vi "All_stats_labels.vi"() -> (0 "No of stats columns":i32[](array[numeric]), 3 "Stats labels":string[](array[string]))   [LabVIEW 2011]
uses:
  Controls/Inst_type.ctl
  Globals/Meas_global.vi
  Globals/Trav_pos_global.vi
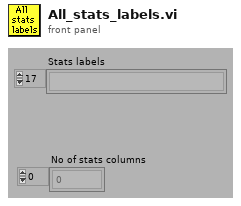
[diagram p1: front panel]
types:
  T1 = typedef "Tunnel_Coordinates.ctl" = enum16{"Work in Tunnel Coordinates", "Work in Model Coordinates"}
  T2 = typedef "Analysis_info_cluster.ctl" = cluster{"Colour":u32, "Inst type":T3, "Inst name":string, "Symbol":string, "Code name":string, "Extra Info":string, "Inst Array":T4, "Index":i32, "Voltage Index":i32, "Extra Titles":string[], "Extra Values":string[], "Eng Values":dbl[], "Time (ms)":dbl[], "TT / Voltage":dbl[], "U":dbl, "u^2":dbl, "u^3":dbl, "u^4":dbl, "Skew_u":dbl, "Kurt_u":dbl, "Sd Error in Mean":dbl, "% u'/U":dbl, "X":dbl, "Y":dbl, "Z":dbl, "Spectra":T5, "Autocorrelation":T5, "Timescale integral to 25%":dbl, "Sd Error in Variance":dbl, "Calib File":path, "Calib Constants":dbl[]}
  T3 = typedef "Inst_type.ctl" = enum16{"Propeller anemometer", "Raw voltage", "Pressure Transducer", "Pitot-static tube", "Preston tube", "Hot wire", "Cross wire 1", "Cross wire 2", "Generic Linear", "Generic Polynomial", "Generic BackPoly", "Fast FID", "Thermocouple", "Cold wire", "Pulsed Wire", "LDA Vel", "LDA Tran time", "LDA Arr time"}
  T4 = typedef "Instrument_Array.ctl" = enum16{"PWA", "LDA", "Analogue"}
  T5 = typedef "XY_Plot_Cluster.ctl" = cluster{"First Name":string, "Second Name":string, "X axis name":string, "Y axis name":string, "X array":dbl[], "Y array":dbl[]}
  T6 = typedef "Analysis_type_cluster.ctl" = cluster{"Analysis type":T7, "Indicies":i32[], "Name":string, "Inst Array":T4, "Info index":i32}
  T7 = typedef "Analysis_type_Enum.ctl" = enum16{"Slow Response", "Fast Response", "Weighted Fast Response", "Fast FID", "Weighted Fast FID", "Cross Wire", "Weighted Cross Wire", "Weighted LDA"}
  T8 = enum16{"Mean only", "2nd Order Stats", "4th Order Stats"}
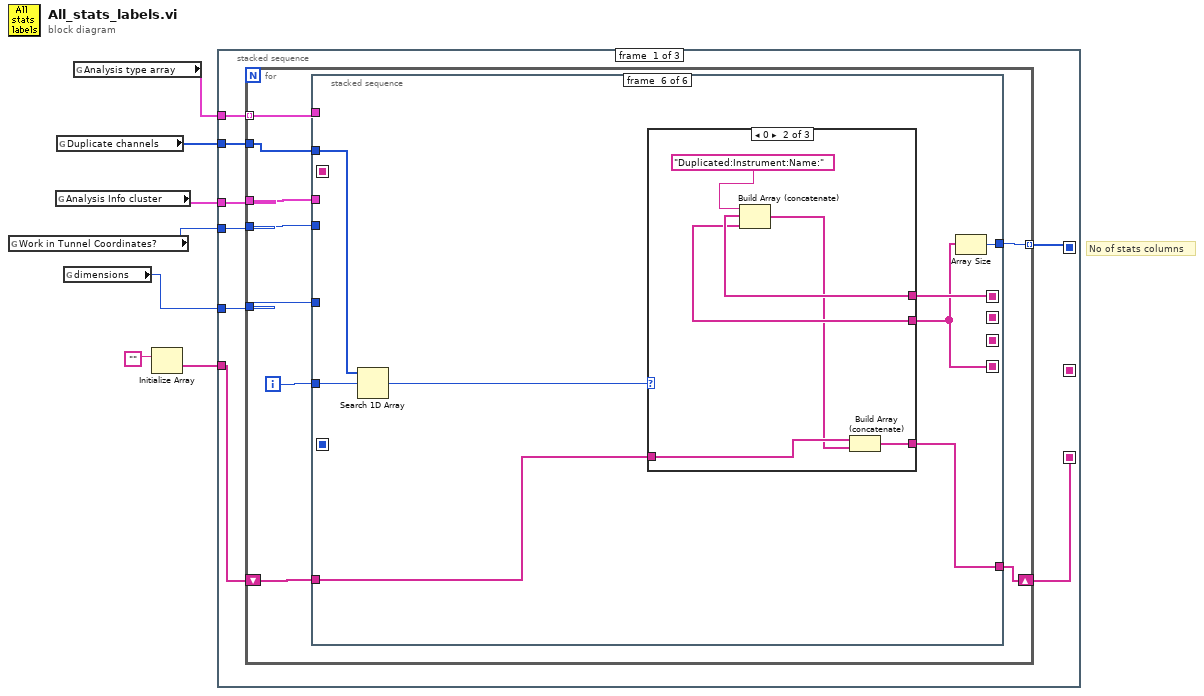
[diagram p0: block diagram]
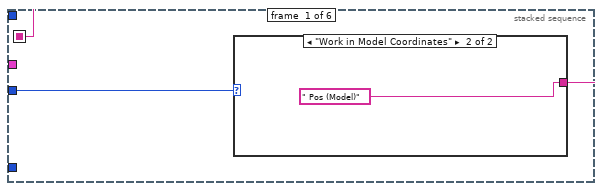
[diagram p2: hidden frame]
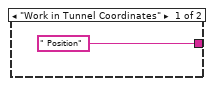
[diagram p3: hidden frame]
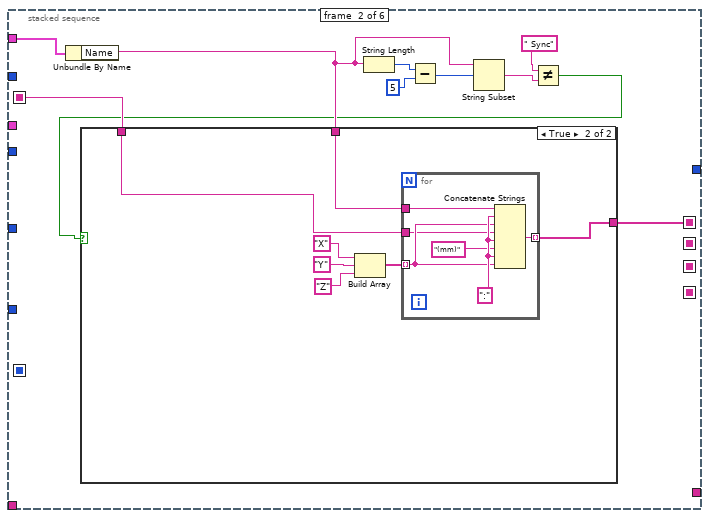
[diagram p4: hidden frame]
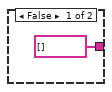
[diagram p5: hidden frame]
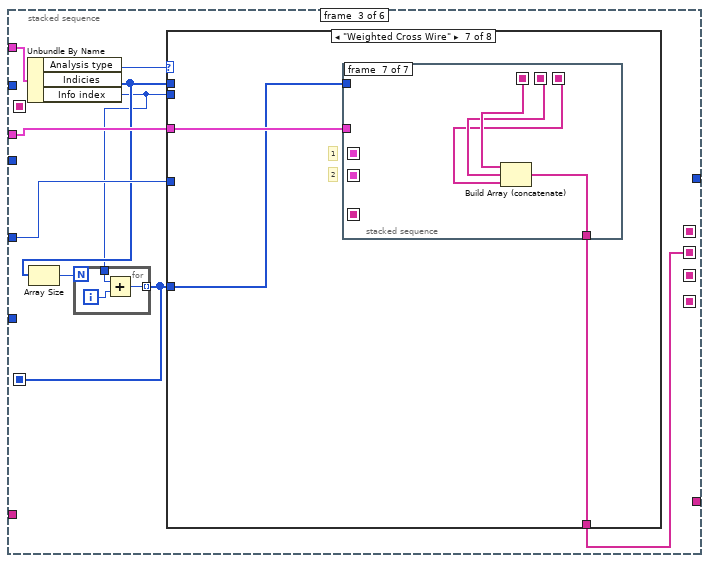
[diagram p6: hidden frame]
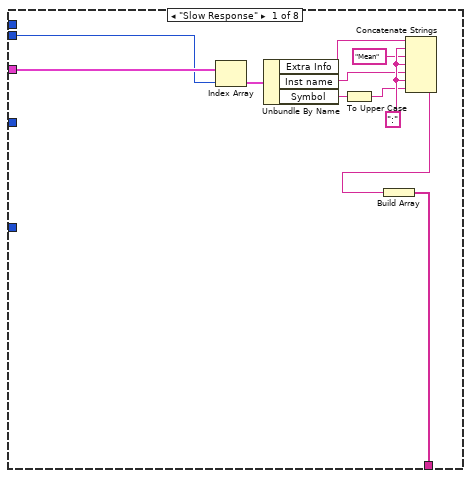
[diagram p7: hidden frame]
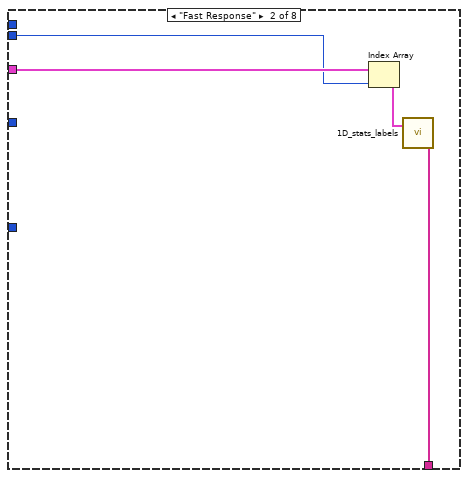
[diagram p8: hidden frame]
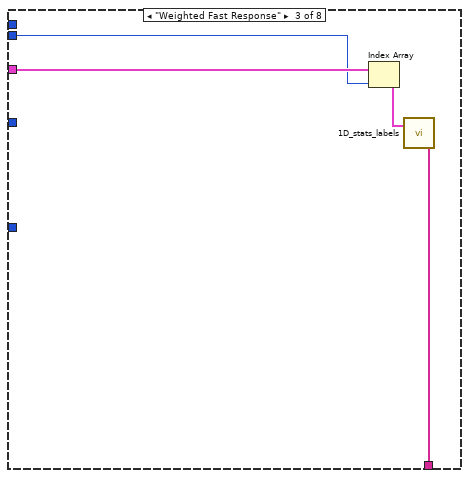
[diagram p9: hidden frame]
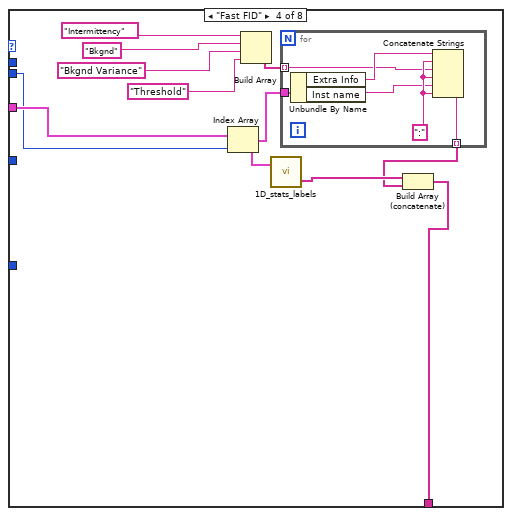
[diagram p10: hidden frame]
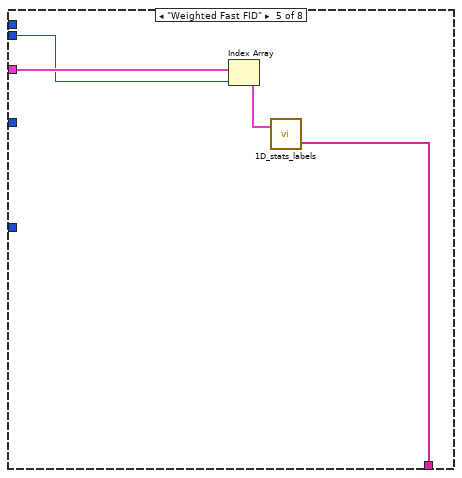
[diagram p11: hidden frame]
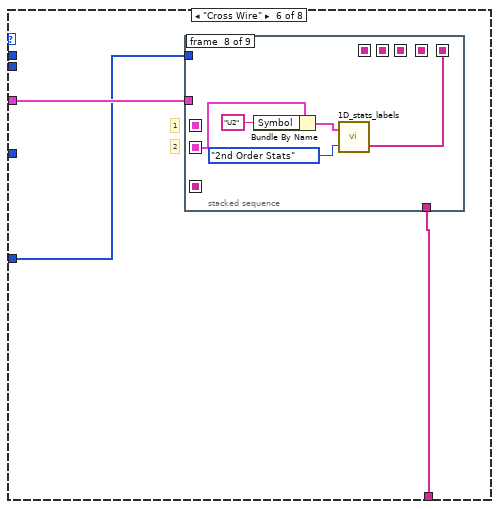
[diagram p12: hidden frame]
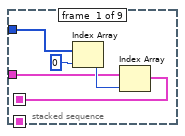
[diagram p13: hidden frame]
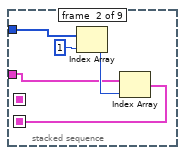
[diagram p14: hidden frame]
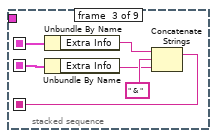
[diagram p15: hidden frame]
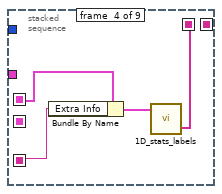
[diagram p16: hidden frame]
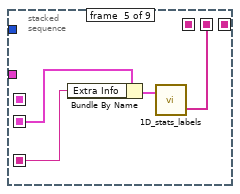
[diagram p17: hidden frame]
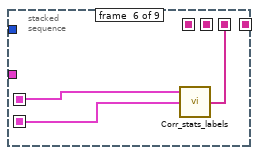
[diagram p18: hidden frame]
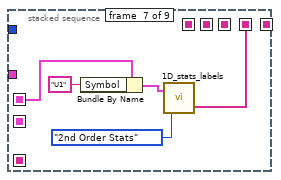
[diagram p19: hidden frame]
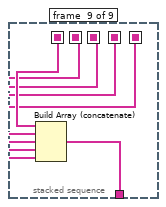
[diagram p20: hidden frame]
diagram:
  # "No of stats columns"
  n1 = global read "Trav_pos_global.vi" "Work in Tunnel Coordinates?"() -> (w2:T1)
  n2 = global read "Meas_global.vi" "Analysis Info cluster"() -> (w3:T2[])
  n3 = global read "Meas_global.vi" "Duplicate channels"() -> (w1:i32[])
  n4 = global read "Meas_global.vi" "dimensions"() -> (w4:enum16{"1D", "2D"})
  n5 = global read "Meas_global.vi" "Analysis type array"() -> (w7:T6[])
  n6 = Initialize Array("") -> (w5:string[])  [unwired: 1 out]
  n7 = stacked-sequence {
    seq-local: [w12 _ _] -> [_ _ w371]
    seq-local: [_ w353 _] -> [_ _ w368]
    seq-local: [w11 _ _] -> [_ _ w369]
    tunnel: w3 -> [w15 w354 _]
    tunnel: w7 -> [w14 _ _]
    tunnel: w5 -> [w10 _ _]
    tunnel: w4 -> [w13 _ _]
    tunnel: w2 -> [w9 _ _]
    tunnel: w1 -> [w8 _ _]
    frame #0 {
      n8 = for {
        shift-right: [w16] -> w12
        shift-left: w10 -> [w17]
        tunnel: w14 -> [w20] mode=indexing
        tunnel: w15 -> [w23]
        tunnel: w13 -> [w24]
        tunnel: [w22] -> w11 mode=indexing
        tunnel: w9 -> [w21]
        tunnel: w8 -> [w18]
        i -> [w19]
        n9 = stacked-sequence {
          seq-local: [_ _ w58 _ _ _] -> [_ _ _ w259 _ _]
          seq-local: [_ w36 _ _ _ _] -> [_ _ _ _ _ w340]
          seq-local: [w25 _ _ _ _ _] -> [_ w37 _ _ _ _]
          seq-local: [_ _ _ w258 _ _] -> [_ _ _ _ w298 _]
          seq-local: [_ _ _ _ w286 _] -> [_ _ _ _ _ w333]
          seq-local: [_ _ w53 _ _ _] -> [_ _ _ w257 w301 _]
          tunnel: w20 -> [_ w38 w61 _ w300 _]
          tunnel: w24 -> [_ _ w59 _ _ _]
          tunnel: w23 -> [_ _ w57 w260 w285 _]
          tunnel: [_ _ _ _ _ w339] -> w22
          tunnel: w21 -> [w26 _ _ _ _ _]
          tunnel: w19 -> [_ _ _ _ _ w338]
          tunnel: w18 -> [_ _ _ _ _ w337]
          tunnel: w17 -> [_ _ _ _ _ w336]
          tunnel: [_ _ _ _ _ w335] -> w16
          frame #0 {
            n10 = case shown="\"Work in Model Coordinates\"" w26 {
              tunnel: [" Position" " Pos (Model)"] -> w25
              frame "Work in Tunnel Coordinates" {
              }
              frame "Work in Model Coordinates" {
              }
            }
          }
          frame #1 {
            n11 = Unbundle By Name(w38) -> ("Name"=w30:string)
            n12 = String Length(string=w30) -> (length=w35:i32)
            n13 = Subtract(x=w35, y=5) -> (x-y=w33:i32)
            n14 = String Subset(string=w30, offset (0)=w33) -> (substring=w31:string)  [unwired: 1 out]
            n15 = Not Equal?(x=" Sync" ("substring"), y=w31) -> (x != y?=w29:bool)
            n16 = case shown="True" w29 {
              tunnel: w30 -> [_ w42]
              tunnel: w37 -> [_ w41]
              tunnel: [string[] [] w40] -> w36
              frame False {
              }
              frame True {
                n17 = Build Array("X", "Y", "Z") -> (w43:string[])
                n18 = for {
                  tunnel: w43 -> [w50] mode=indexing
                  tunnel: w42 -> [w52]
                  tunnel: [w48] -> w40 mode=indexing
                  tunnel: w41 -> [w47]
                  w51 = ":" ("Substring")
                  n19 = Concatenate Strings(w52, w51, w50, w47, w51, "(mm)", w51, w50) -> (w48:string)
                }
              }
            }
          }
          frame #2 {
            n20 = Unbundle By Name(w61) -> ("Analysis type"=w60:T7, "Indicies"=w55:i32[], "Info index"=w54:i32)
            n21 = Array Size(array=w55) -> (size(s)=w56:i32)
            n22 = for {
              N: w56 -> [_]
              tunnel: w54 -> [w63]
              tunnel: [w62] -> w53 mode=indexing
              i -> [w64]
              n23 = Add(x=w63, y=w64) -> (x+y=w62:i32)
            }
            n24 = case shown="\"Weighted Cross Wire\"" w60 {
              tunnel: w55 -> [_ _ _ _ _ _ _ _]
              tunnel: [w66 w78 w82 w91 w102 w107 w153 w188] -> w58
              tunnel: w59 -> [_ _ _ _ _ _ _ w187]
              tunnel: w57 -> [w75 w77 w81 w89 w104 w106 w152 w186]
              tunnel: w54 -> [w65 w76 w80 w84 w101 _ _ _]
              tunnel: w53 -> [_ _ _ _ _ w105 w151 w185]
              frame "Slow Response" {
                w74 = ":" ("Substring")
                n25 = Index Array(array=w75, index=w65) -> (element=w68:T2)
                n26 = Unbundle By Name(w68) -> ("Extra Info"=w73:string, "Inst name"=w71:string, "Symbol"=w70:string)
                n27 = To Upper Case(1:w70) -> (0:w69:string)
                n28 = Concatenate Strings(w73, w74, "Mean", w74, w71, w74, w69) -> (w67:string)
                n29 = Build Array(w67) -> (w66:string[])
              }
              frame "Fast Response" {
                n30 = Index Array(array=w77, index=w76) -> (element=w79:T2)
                n31 = call "1D_stats_labels.vi"("Analysis Info Cluster"=w79) -> ("Output"=w78:string[])  [unwired: 1 in, 1 out]
              }
              frame "Weighted Fast Response" {
                n32 = Index Array(array=w81, index=w80) -> (element=w83:T2)
                n33 = call "1D_stats_labels.vi"("Analysis Info Cluster"=w83) -> ("Output"=w82:string[])  [unwired: 1 in, 1 out]
              }
              frame "Fast FID" {
                n34 = Index Array(array=w89, index=w84) -> (element=w94:T2)
                n35 = Build Array("Intermittency", "Bkgnd", "Bkgnd Variance", "Threshold") -> (w90:string[])
                n36 = call "1D_stats_labels.vi"("Analysis Info Cluster"=w94) -> ("Output"=w93:string[])  [unwired: 1 in, 1 out]
                n37 = for {
                  tunnel: w94 -> [w97]
                  tunnel: [w96] -> w92 mode=indexing
                  tunnel: w90 -> [w95] mode=indexing
                  w100 = ":" ("Substring")
                  n38 = Unbundle By Name(w97) -> ("Extra Info"=w99:string, "Inst name"=w98:string)
                  n39 = Concatenate Strings(w99, w100, w95, w100, w98, w100) -> (w96:string)
                }
                n40 = Build Array (concatenate)(w93, w92) -> (w91:string[])
              }
              frame "Weighted Fast FID" {
                n41 = Index Array(array=w104, index=w101) -> (element=w103:T2)
                n42 = call "1D_stats_labels.vi"("Analysis Info Cluster"=w103) -> ("Output"=w102:string[])  [unwired: 1 in, 1 out]
              }
              frame "Cross Wire" {
                # "2"
                # "1"
                n43 = stacked-sequence {
                  seq-local: [_ _ _ w127 _ _ _ _ _] -> [_ _ _ _ _ _ _ _ w150]
                  seq-local: [_ _ _ _ w131 _ _ _ _] -> [_ _ _ _ _ _ _ _ w149]
                  seq-local: [_ _ _ _ _ w134 _ _ _] -> [_ _ _ _ _ _ _ _ w148]
                  seq-local: [_ _ _ _ _ _ w139 _ _] -> [_ _ _ _ _ _ _ _ w147]
                  seq-local: [_ _ _ _ _ _ _ w144 _] -> [_ _ _ _ _ _ _ _ w146]
                  seq-local: [w108 _ _ _ _ _ _ _ _] -> [_ _ w123 w126 _ w133 w137 _ _]
                  seq-local: [_ w113 _ _ _ _ _ _ _] -> [_ _ w122 _ w129 w132 _ w141 _]
                  seq-local: [_ _ w121 _ _ _ _ _ _] -> [_ _ _ w125 w128 _ _ _ _]
                  tunnel: [_ _ _ _ _ _ _ _ w145] -> w107
                  tunnel: w105 -> [w110 w115 _ _ _ _ _ _ _]
                  tunnel: w106 -> [w109 w114 _ _ _ _ _ _ _]
                  frame #0 {
                    n44 = Index Array(array=w110, index=0) -> (element=w112:i32)
                    n45 = Index Array(array=w109, index=w112) -> (element=w108:T2)
                  }
                  frame #1 {
                    n46 = Index Array(array=w115, index=1) -> (element=w117:i32)
                    n47 = Index Array(array=w114, index=w117) -> (element=w113:T2)
                  }
                  frame #2 {
                    n48 = Unbundle By Name(w123) -> ("Extra Info"=w118:string)
                    n49 = Unbundle By Name(w122) -> ("Extra Info"=w119:string)
                    n50 = Concatenate Strings(w118, " & ", w119) -> (w121:string)
                  }
                  frame #3 {
                    n51 = Bundle By Name(cluster=w126, "Extra Info"=w125) -> (w124:T2)
                    n52 = call "1D_stats_labels.vi"("Analysis Info Cluster"=w124) -> ("Output"=w127:string[])  [unwired: 1 in, 1 out]
                  }
                  frame #4 {
                    n53 = Bundle By Name(cluster=w129, "Extra Info"=w128) -> (w130:T2)
                    n54 = call "1D_stats_labels.vi"("Analysis Info Cluster"=w130) -> ("Output"=w131:string[])  [unwired: 1 in, 1 out]
                  }
                  frame #5 {
                    n55 = call "Corr_stats_labels.vi"("Inst 2 Units"=w132, "Inst 1 Units"=w133) -> ("Output"=w134:string[])  [unwired: 1 in]
                  }
                  frame #6 {
                    n56 = Bundle By Name(cluster=w137, "Symbol"="U1") -> (w136:T2)
                    n57 = call "1D_stats_labels.vi"("Mode selector"=T8."2nd Order Stats", "Analysis Info Cluster"=w136) -> ("Output"=w139:string[])  [unwired: 1 out]
                  }
                  frame #7 {
                    n58 = Bundle By Name(cluster=w141, "Symbol"="U2") -> (w140:T2)
                    n59 = call "1D_stats_labels.vi"("Mode selector"=T8."2nd Order Stats", "Analysis Info Cluster"=w140) -> ("Output"=w144:string[])  [unwired: 1 out]
                  }
                  frame #8 {
                    n60 = Build Array (concatenate)(w150, w149, w148, w147, w146) -> (w145:string[])
                  }
                }
              }
              frame "Weighted Cross Wire" {
                # "2"
                # "1"
                n61 = stacked-sequence {
                  seq-local: [_ _ _ w173 _ _ _] -> [_ _ _ _ _ _ w184]
                  seq-local: [_ _ _ _ w177 _ _] -> [_ _ _ _ _ _ w183]
                  seq-local: [_ _ _ _ _ w180 _] -> [_ _ _ _ _ _ w182]
                  seq-local: [w154 _ _ _ _ _ _] -> [_ _ w169 w172 _ w179 _]
                  seq-local: [_ w159 _ _ _ _ _] -> [_ _ w168 _ w175 w178 _]
                  seq-local: [_ _ w167 _ _ _ _] -> [_ _ _ w171 w174 _ _]
                  tunnel: [_ _ _ _ _ _ w181] -> w153
                  tunnel: w151 -> [w156 w161 _ _ _ _ _]
                  tunnel: w152 -> [w155 w160 _ _ _ _ _]
                  frame #0 {
                    n62 = Index Array(array=w156, index=0) -> (element=w158:i32)
                    n63 = Index Array(array=w155, index=w158) -> (element=w154:T2)
                  }
                  frame #1 {
                    n64 = Index Array(array=w161, index=1) -> (element=w163:i32)
                    n65 = Index Array(array=w160, index=w163) -> (element=w159:T2)
                  }
                  frame #2 {
                    n66 = Unbundle By Name(w169) -> ("Extra Info"=w164:string)
                    n67 = Unbundle By Name(w168) -> ("Extra Info"=w165:string)
                    n68 = Concatenate Strings(w164, " & ", w165) -> (w167:string)
                  }
                  frame #3 {
                    n69 = Bundle By Name(cluster=w172, "Extra Info"=w171) -> (w170:T2)
                    n70 = call "1D_stats_labels.vi"("Analysis Info Cluster"=w170) -> ("Output"=w173:string[])  [unwired: 1 in, 1 out]
                  }
                  frame #4 {
                    n71 = Bundle By Name(cluster=w175, "Extra Info"=w174) -> (w176:T2)
                    n72 = call "1D_stats_labels.vi"("Analysis Info Cluster"=w176) -> ("Output"=w177:string[])  [unwired: 1 in, 1 out]
                  }
                  frame #5 {
                    n73 = call "Corr_stats_labels.vi"("Inst 2 Units"=w178, "Inst 1 Units"=w179) -> ("Output"=w180:string[])  [unwired: 1 in]
                  }
                  frame #6 {
                    n74 = Build Array (concatenate)(w184, w183, w182) -> (w181:string[])
                  }
                }
              }
              frame "Weighted LDA" {
                n75 = case shown="\"2D\"" w187 {
                  tunnel: [w191 w216] -> w188
                  tunnel: w185 -> [w190 w215]
                  tunnel: w186 -> [w189 w214]
                  frame "1D" {
                    n76 = stacked-sequence {
                      seq-local: [w193 _ _] -> [_ _ w213]
                      seq-local: [_ w199 _] -> [_ _ w212]
                      tunnel: [_ _ w211] -> w191
                      tunnel: w190 -> [w194 w203 _]
                      tunnel: w189 -> [w192 w198 _]
                      frame #0 {
                        n77 = Index Array(array=w194, index=0) -> (element=w196:i32)
                        n78 = Index Array(array=w192, index=w196) -> (element=w197:T2)
                        n79 = call "1D_stats_labels.vi"("Analysis Info Cluster"=w197) -> ("Output"=w193:string[])  [unwired: 1 in, 1 out]
                      }
                      frame #1 {
                        n80 = Split 1D Array(array=w203, index=2) -> (second subarray=w201:i32[])  [unwired: 1 out]
                        n81 = for {
                          tunnel: w201 -> [w209] mode=indexing
                          shift-right: [w206] -> w199
                          shift-left: string[] [] -> [w208]
                          tunnel: w198 -> [w205]
                          n82 = Index Array(array=w205, index=w209) -> (element=w210:T2)
                          n83 = call "1D_stats_labels.vi"("Mode selector"=T8."Mean only", "Analysis Info Cluster"=w210) -> ("Output"=w207:string[])  [unwired: 1 out]
                          n84 = Build Array (concatenate)(w208, w207) -> (w206:string[])
                        }
                      }
                      frame #2 {
                        n85 = Build Array (concatenate)(w213, w212) -> (w211:string[])
                      }
                    }
                  }
                  frame "2D" {
                    n86 = stacked-sequence {
                      seq-local: [w218 _ _ _ _] -> [_ _ _ _ w255]
                      seq-local: [_ w224 _ _ _] -> [_ _ _ _ w254]
                      seq-local: [_ _ w230 _ _] -> [_ _ _ _ w253]
                      seq-local: [_ _ _ w239 _] -> [_ _ _ _ w252]
                      tunnel: [_ _ _ _ w251] -> w216
                      tunnel: w215 -> [w219 w225 w233 w243 _]
                      tunnel: w214 -> [w217 w223 w229 w238 _]
                      frame #0 {
                        n87 = Index Array(array=w219, index=0) -> (element=w221:i32)
                        n88 = Index Array(array=w217, index=w221) -> (element=w222:T2)
                        n89 = call "1D_stats_labels.vi"("Analysis Info Cluster"=w222) -> ("Output"=w218:string[])  [unwired: 1 in, 1 out]
                      }
                      frame #1 {
                        n90 = Index Array(array=w225, index=1) -> (element=w227:i32)
                        n91 = Index Array(array=w223, index=w227) -> (element=w228:T2)
                        n92 = call "1D_stats_labels.vi"("Analysis Info Cluster"=w228) -> ("Output"=w224:string[])  [unwired: 1 in, 1 out]
                      }
                      frame #2 {
                        n93 = Index Array(array=w233, index=0) -> (element=w236:i32)
                        n94 = Index Array(array=w233, index=1) -> (element=w232:i32)
                        n95 = Index Array(array=w229, index=w236) -> (element=w237:T2)
                        n96 = Index Array(array=w229, index=w232) -> (element=w231:T2)
                        n97 = call "Corr_stats_labels.vi"("Inst 2 Units"=w231, "Inst 1 Units"=w237) -> ("Output"=w230:string[])  [unwired: 1 in]
                      }
                      frame #3 {
                        n98 = Split 1D Array(array=w243, index=2) -> (second subarray=w241:i32[])  [unwired: 1 out]
                        n99 = for {
                          tunnel: w241 -> [w249] mode=indexing
                          shift-right: [w246] -> w239
                          shift-left: string[] [] -> [w248]
                          tunnel: w238 -> [w245]
                          n100 = Index Array(array=w245, index=w249) -> (element=w250:T2)
                          n101 = call "1D_stats_labels.vi"("Mode selector"=T8."Mean only", "Analysis Info Cluster"=w250) -> ("Output"=w247:string[])  [unwired: 1 out]
                          n102 = Build Array (concatenate)(w248, w247) -> (w246:string[])
                        }
                      }
                      frame #4 {
                        n103 = Build Array (concatenate)(w255, w254, w253, w252) -> (w251:string[])
                      }
                    }
                  }
                }
              }
            }
          }
          frame #3 {
            n104 = global read "Meas_global.vi" "Timescales (s)"() -> (w256:dbl[])
            n105 = for {
              tunnel: w256 -> [w264]
              tunnel: w257 -> [w261] mode=indexing
              shift-right: [w265] -> w258
              shift-left: w259 -> [w267]
              tunnel: w260 -> [w266]
              n106 = Index Array(array=w264, index=w261) -> (element=w263:dbl)
              n107 = Not A Number/Path/Refnum?(number/path/refnum=w263) -> (NaN/Path/Refnum?=w262:bool)
              n108 = case shown="False" w262 {
                tunnel: w267 -> [w280 w281]
                tunnel: [w279 w281] -> w265
                tunnel: w261 -> [w277 _]
                tunnel: w266 -> [w278 _]
                frame False {
                  n109 = Index Array(array=w278, index=w277) -> (element=w276:T2)
                  n110 = Unbundle By Name(w276) -> ("Inst name"=w272:string)
                  n111 = Format Into String(format string="%s:Standard Error:in Mean:Not %%", w272) -> (resulting string=w274:string)  [unwired: 2 in, 1 out]
                  n112 = Format Into String(format string="%s:Standard Error:in Variance:Not %%", w272) -> (resulting string=w270:string)  [unwired: 2 in, 1 out]
                  n113 = Format Into String(format string="%s:Timescale Estimate:Integrated to 25%%:(s)", w272) -> (resulting string=w268:string)  [unwired: 2 in, 1 out]
                  n114 = Build Array(w274, w270, w268) -> (w273:string[])
                  n115 = Build Array (concatenate)(w280, w273) -> (w279:string[])
                }
                frame True {
                }
              }
            }
          }
          frame #4 {
            n116 = Unbundle By Name(w300) -> ("Name"=w296:string)
            n117 = Index Array(array=w301, index=0 ("Index")) -> (element=w295:i32)
            n118 = Index Array(array=w285, index=w295) -> (element=w303:T2)
            n119 = Unbundle By Name(w303) -> ("Code name"=w289:string, "Inst type"=w293:T3, "Extra Titles"=w283:string[], "Inst name"=w284:string)
            n120 = Format Into String(format string="%s:Calibration:Filename" ("Format String"), w296) -> (resulting string=w297:string)  [unwired: 2 in, 1 out]
            n121 = for {
              tunnel: w284 -> [w307]
              tunnel: w283 -> [w305] mode=indexing
              tunnel: [w304] -> w282 mode=indexing
              n122 = Concatenate Strings(w307, ":" ("string"), w305) -> (w304:string)
            }
            n123 = Match Pattern(string=w289, regular expression="Derived") -> (offset past match=w290:i32)  [unwired: 4 out]
            n124 = Greater Or Equal To 0?(x=w290) -> (x >= 0?=w288:bool)
            n125 = Select(t=Inst_type."LDA Vel" ("Inst type"), s=w288, f=w293) -> (s? t:f=w292:T3)
            n126 = case shown="\"Generic Linear\", Default" w292 {
              tunnel: [w310 w313 w316 w322 w325 w329 w331 w332] -> w287
              tunnel: w298 -> [w309 w312 w315 w324 w327 w330 w331 w332]
              tunnel: w297 -> [w308 w311 w314 w323 w326 w328 _ _]
              tunnel: w296 -> [_ _ _ w319 _ _ _ _]
              frame "Propeller anemometer" {
                n127 = Build Array (concatenate)(w309, w308) -> (w310:string[])
              }
              frame "Preston tube" {
                n128 = Build Array (concatenate)(w312, w311) -> (w313:string[])
              }
              frame "Pressure Transducer" {
                n129 = Build Array (concatenate)(w315, w314) -> (w316:string[])
              }
              frame "Generic Linear", Default {
                n130 = Format Into String(format string="%s:Calibration:Drift:%%" ("Format String"), w319) -> (resulting string=w318:string)  [unwired: 2 in, 1 out]
                n131 = Format Into String(format string="%s:Calibration:Interval:Minutes" ("Format String"), w319) -> (resulting string=w317:string)  [unwired: 2 in, 1 out]
                n132 = Build Array (concatenate)(w324, w323, w318, w317) -> (w322:string[])
              }
              frame "Pulsed Wire" {
                n133 = Build Array (concatenate)(w327, w326) -> (w325:string[])
              }
              frame "Pitot-static tube" {
                n134 = Build Array (concatenate)(w330, w328) -> (w329:string[])
              }
              frame "Raw voltage" {
              }
              frame "LDA Vel" {
              }
            }
            n135 = Build Array (concatenate)(w287, w282) -> (w286:string[])
          }
          frame #5 {
            n136 = Search 1D Array(1D array=w337, element=w338) -> (index of element=w334:i32)  [unwired: 1 out]
            n137 = case shown="0" w334 {
              tunnel: w340 -> [w345 w351 _]
              tunnel: w333 -> [w344 w350 _]
              tunnel: w336 -> [w343 w349 w352]
              tunnel: [w342 w346 w352] -> w335
              frame -1 {
                n138 = Build Array (concatenate)(w345, w344) -> (w341:string[])
                n139 = Build Array (concatenate)(w343, w341) -> (w342:string[])
              }
              frame 0 {
                n140 = Build Array (concatenate)("Duplicated:Instrument:Name:", w351, w350) -> (w348:string[])
                n141 = Build Array (concatenate)(w349, w348) -> (w346:string[])
              }
              frame 1, Default {
              }
            }
            n142 = Array Size(array=w333) -> (size(s)=w339:i32)
          }
        }
      }
    }
    frame #1 {
      n143 = global read "Meas_global.vi" "correlate"() -> (w355:i32[][])
      n144 = for {
        shift-right: [w366] -> w353
        shift-left: string[] [] -> [w367]
        tunnel: w355 -> [w360] mode=indexing
        tunnel: w354 -> [w359]
        n145 = Index Array(array=w360, index=0) -> (element=w364:i32)
        n146 = Index Array(array=w360, index=1) -> (element=w362:i32)
        n147 = Index Array(array=w359, index=w364) -> (element=w358:T2)
        n148 = Index Array(array=w359, index=w362) -> (element=w357:T2)
        n149 = call "Corr_stats_labels.vi"("Inst 2 Units"=w357, "Inst 1 Units"=w358) -> ("Output"=w365:string[])  [unwired: 1 in]
        n150 = Build Array (concatenate)(w367, w365) -> (w366:string[])
      }
    }
    frame #2 {
      n151 = Build Array (concatenate)(w371, w368) -> (→"Stats labels":string[])
      "No of stats columns" <- w369
    }
  }
